vi "fpga_start.vi"(8 "error in":errorcluster, 10 "Timeout (ms)":u32=1000, 11 "FPGA VI Reference in":T1) -> (0 "error out":errorcluster, 2 "Timed out?":bool, 3 "FPGA VI Reference out":T1)   [LabVIEW 2011, in "Fiberscope_library.lvlib"]
uses:
  Fiberscope_library.lvlib
  typedefs/fpga_main_spiral_fpga_ref.ctl
  <vilib>/Utility/error.llb/Error Cluster From Error Code.vi
  <vilib>/rvi/errors/niLvFpgaAdjustHostInterfaceError.vi
  <vilib>/rvi/interface/nirviReadWriteControl/nirviReadWriteControl.xnode
  FPGA Bitfiles/FiberscopeRK1107_FPGATarget_fpgamainspiral_0DF2A7CB.lvbitx
  NiFpgaLv.dll
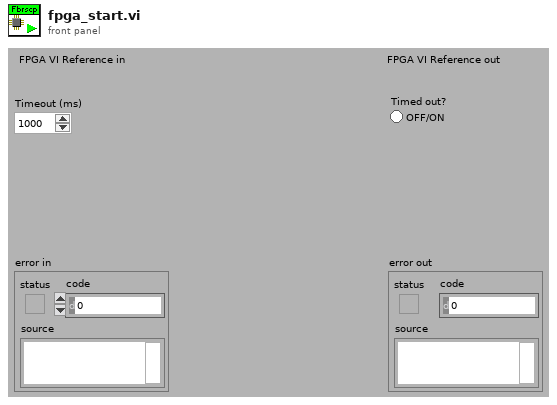
[diagram p1: front panel]
types:
  T1 = typedef "Fiberscope_library.lvlib/fpga_main_spiral_fpga_ref.ctl" = refnum<k20>
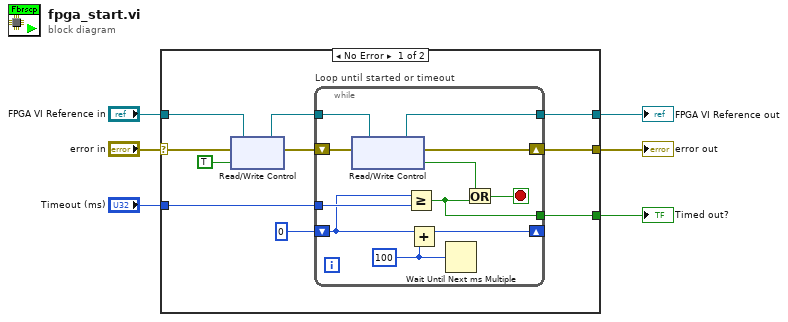
[diagram p0: block diagram]
diagram:
  n1 = case shown="No Error" "error in" {
    selector: "error in" -> [w15 w29]
    tunnel: [w10 w29] -> w5
    tunnel: "FPGA VI Reference in" -> [w16 w28]
    tunnel: [w11 w28] -> w3
    tunnel: "Timeout (ms)" -> [w9 _]
    tunnel: [w7 _] -> w1
    frame No Error {
      n2 = xnode "Read/Write Control"("FPGA VI Reference In"=w16, "error in"=w15, "Scan"=TRUE) -> ("FPGA VI Reference Out"=w12:T1, "error out"=w13:errorcluster)
      n3 = while "Loop until started or timeout" {
        shift-right: [w25] -> w10
        shift-left: w13 -> [w27]
        tunnel: w12 -> [w26]
        tunnel: [w23] -> w11
        tunnel: w9 -> [w21]
        shift-right: [w19] -> _
        shift-left: u32 0 -> [w20]
        tunnel: [w17] -> w7
        stop <- w24 stop-if-true
        w18 = u32 100 ("millisecond multiple")
        n4 = xnode "Read/Write Control"("FPGA VI Reference In"=w26, "error in"=w27) -> ("FPGA VI Reference Out"=w23:T1, "error out"=w25:errorcluster, "Scanning?"=w22:bool)
        n5 = Greater Or Equal?(x=w20, y=w21) -> (x >= y?=w17:bool)
        n6 = Add(x=w20, y=w18) -> (x+y=w19:u32)
        n7 = Wait Until Next ms Multiple(millisecond multiple=w18) -> ()  [unwired: 1 out]
        n8 = Or(x=w22, y=w17) -> (x .or. y?=w24:bool)
      }
    }
    frame Error {
    }
  }
  "error out" <- w5
  "FPGA VI Reference out" <- w3
  "Timed out?" <- w1
